vi "ExecuteMenuCommand.vi"(0 "reference":refnum<class "ClassRelationshipEdge.lvclass">, 1 "Command":string, 5 "error in (no error)":errorcluster) -> (14 "reference out":refnum<class "ClassRelationshipEdge.lvclass">, 15 "EditorAction":T1, 19 "error out":errorcluster)   [LabVIEW 2016, in "ClassRelationshipEdge.lvclass"]
uses:
  <resource>/Framework/Providers/Open_GDS/UML/ClassRelationshipEdge_class/ClassRelationshipEdge.lvclass
  <resource>/Framework/Providers/Open_GDS/UML/UMLEditor/UMLEditor EditorActionType.ctl
  <resource>/Framework/Providers/Open_GDS/UML/BentStyle_class/BentStyleType.ctl
  <resource>/Framework/Providers/Open_GDS/UML/BentStyle_class/BentStyle.lvclass
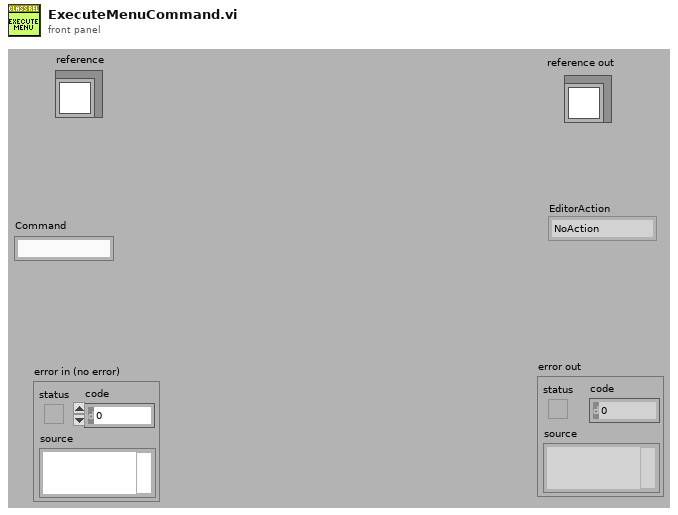
[diagram p1: front panel]
types:
  T1 = typedef "UMLEditor EditorActionType.ctl" = enum16{"NoAction", "Repaint", "ExecuteCommand"}
  T2 = typedef "BentStyle.lvclass/BentStyleType.ctl" = enum16{"STRAIGHT", "HV", "VH", "HVH", "VHV", "ARC"}
  T3 = typedef "ClassRelationshipEdge.lvclass/ObjectAttributes.ctl" = cluster{"bentStyleRef":refnum<class "BentStyle.lvclass">, "startConnectionOffset":cluster{"x":i32, "y":i32}, "endConnectionOffset":cluster{"x":i32, "y":i32}, "MidLineOffset":cluster{"x":i32, "y":i32}, "DepClass":T4}
  T4 = typedef "ReversedEngineering_ViDependencyDetailsType.ctl" = cluster{"ThisVIs/Ctls":path[], "Dependent_VIs/Ctls":path[]}
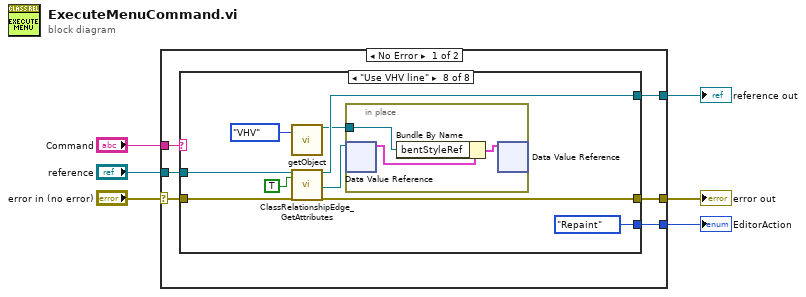
[diagram p0: block diagram]
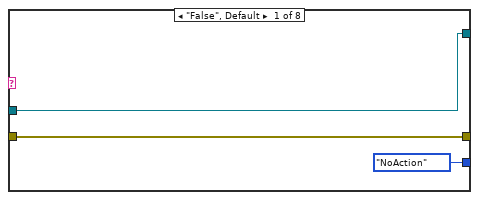
[diagram p2: hidden frame]
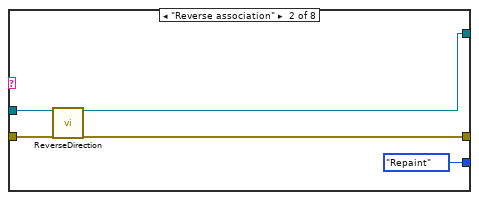
[diagram p3: hidden frame]
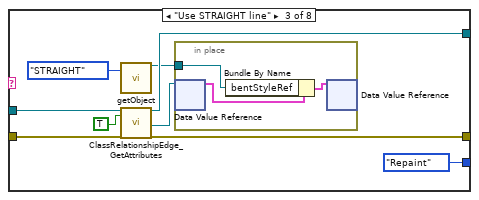
[diagram p4: hidden frame]
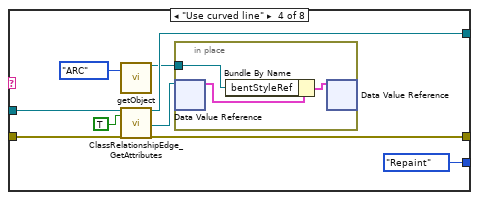
[diagram p5: hidden frame]
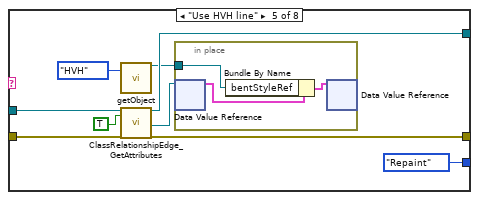
[diagram p6: hidden frame]
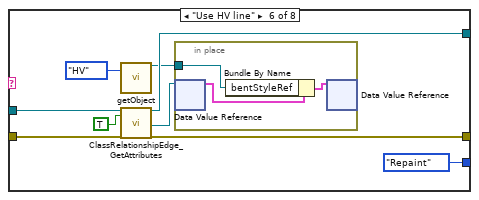
[diagram p7: hidden frame]
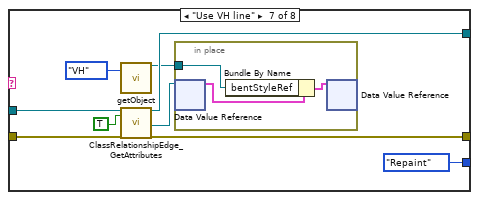
[diagram p8: hidden frame]
diagram:
  n1 = case shown="No Error" "error in (no error)" {
    selector: "error in (no error)" -> [w10 w93]
    tunnel: "reference" -> [w11 w94]
    tunnel: [w9 w93] -> w4
    tunnel: [w7 w94] -> w3
    tunnel: [w8 _] -> w2
    tunnel: "Command" -> [w12 _]
    frame No Error {
      n2 = case shown="\"Use VHV line\"" w12 {
        tunnel: w11 -> [w13 w20 w28 w40 w52 w64 w76 w88]
        tunnel: w10 -> [w14 w19 w27 w39 w51 w63 w75 w87]
        tunnel: [w14 w18 w26 w38 w50 w62 w74 w86] -> w9
        tunnel: [UMLEditor_EditorActionType."NoAction" ("EditorAction") UMLEditor_EditorActionType."Repaint" ("EditorAction") UMLEditor_EditorActionType."Repaint" ("EditorAction") UMLEditor_EditorActionType."Repaint" ("EditorAction") UMLEditor_EditorActionType."Repaint" ("EditorAction") UMLEditor_EditorActionType."Repaint" ("EditorAction") UMLEditor_EditorActionType."Repaint" ("EditorAction") UMLEditor_EditorActionType."Repaint" ("EditorAction")] -> w8
        tunnel: [w13 w16 w25 w37 w49 w61 w73 w85] -> w7
        frame "False", Default {
        }
        frame "Reverse association" {
          n3 = call-dynamic "ReverseDirection.vi"("reference"=w20, "error in (no error)"=w19) -> ("reference out"=w16:refnum<class "ClassRelationshipEdge.lvclass">, "error out"=w18:errorcluster)  [unwired: 16 in]
        }
        frame "Use STRAIGHT line" {
          n4 = call <resource>:"getObject.vi"("bentStyle"=BentStyleType."STRAIGHT") -> ("reference out"=w21:refnum<class "BentStyle.lvclass">)  [unwired: 1 in, 17 out]
          n5 = call <resource>:"ClassRelationshipEdge_GetAttributes.vi"("reference in"=w28, "OnlyGetDvrReference(False)"=TRUE, "error in (no error)"=w27) -> ("reference out"=w25:refnum<class "ClassRelationshipEdge.lvclass">, "DataRef"=w22:refnum<data-value>, "error out"=w26:errorcluster)  [unwired: 13 in, 1 out]
          n6 = in-place {
            in-place-border: w21 -> [w31]
            n7 = in-place-dvr #1(w22) -> (w32:T3)  [unwired: 1 out]
            n8 = Bundle By Name(cluster=w32, "bentStyleRef"=w31) -> (w30:T3)
            n9 = in-place-dvr #1(w30) -> ()  [unwired: 2 out]
          }
        }
        frame "Use curved line" {
          n10 = call <resource>:"getObject.vi"("bentStyle"=BentStyleType."ARC") -> ("reference out"=w33:refnum<class "BentStyle.lvclass">)  [unwired: 1 in, 17 out]
          n11 = call <resource>:"ClassRelationshipEdge_GetAttributes.vi"("reference in"=w40, "OnlyGetDvrReference(False)"=TRUE, "error in (no error)"=w39) -> ("reference out"=w37:refnum<class "ClassRelationshipEdge.lvclass">, "DataRef"=w34:refnum<data-value>, "error out"=w38:errorcluster)  [unwired: 13 in, 1 out]
          n12 = in-place {
            in-place-border: w33 -> [w43]
            n13 = in-place-dvr #2(w34) -> (w44:T3)  [unwired: 1 out]
            n14 = Bundle By Name(cluster=w44, "bentStyleRef"=w43) -> (w42:T3)
            n15 = in-place-dvr #2(w42) -> ()  [unwired: 2 out]
          }
        }
        frame "Use HVH line" {
          n16 = call <resource>:"getObject.vi"("bentStyle"=BentStyleType."HVH") -> ("reference out"=w45:refnum<class "BentStyle.lvclass">)  [unwired: 1 in, 17 out]
          n17 = call <resource>:"ClassRelationshipEdge_GetAttributes.vi"("reference in"=w52, "OnlyGetDvrReference(False)"=TRUE, "error in (no error)"=w51) -> ("reference out"=w49:refnum<class "ClassRelationshipEdge.lvclass">, "DataRef"=w46:refnum<data-value>, "error out"=w50:errorcluster)  [unwired: 13 in, 1 out]
          n18 = in-place {
            in-place-border: w45 -> [w55]
            n19 = in-place-dvr #3(w46) -> (w56:T3)  [unwired: 1 out]
            n20 = Bundle By Name(cluster=w56, "bentStyleRef"=w55) -> (w54:T3)
            n21 = in-place-dvr #3(w54) -> ()  [unwired: 2 out]
          }
        }
        frame "Use HV line" {
          n22 = call <resource>:"getObject.vi"("bentStyle"=BentStyleType."HV") -> ("reference out"=w57:refnum<class "BentStyle.lvclass">)  [unwired: 1 in, 17 out]
          n23 = call <resource>:"ClassRelationshipEdge_GetAttributes.vi"("reference in"=w64, "OnlyGetDvrReference(False)"=TRUE, "error in (no error)"=w63) -> ("reference out"=w61:refnum<class "ClassRelationshipEdge.lvclass">, "DataRef"=w58:refnum<data-value>, "error out"=w62:errorcluster)  [unwired: 13 in, 1 out]
          n24 = in-place {
            in-place-border: w57 -> [w67]
            n25 = in-place-dvr #4(w58) -> (w68:T3)  [unwired: 1 out]
            n26 = Bundle By Name(cluster=w68, "bentStyleRef"=w67) -> (w66:T3)
            n27 = in-place-dvr #4(w66) -> ()  [unwired: 2 out]
          }
        }
        frame "Use VH line" {
          n28 = call <resource>:"getObject.vi"("bentStyle"=BentStyleType."VH") -> ("reference out"=w69:refnum<class "BentStyle.lvclass">)  [unwired: 1 in, 17 out]
          n29 = call <resource>:"ClassRelationshipEdge_GetAttributes.vi"("reference in"=w76, "OnlyGetDvrReference(False)"=TRUE, "error in (no error)"=w75) -> ("reference out"=w73:refnum<class "ClassRelationshipEdge.lvclass">, "DataRef"=w70:refnum<data-value>, "error out"=w74:errorcluster)  [unwired: 13 in, 1 out]
          n30 = in-place {
            in-place-border: w69 -> [w79]
            n31 = in-place-dvr #5(w70) -> (w80:T3)  [unwired: 1 out]
            n32 = Bundle By Name(cluster=w80, "bentStyleRef"=w79) -> (w78:T3)
            n33 = in-place-dvr #5(w78) -> ()  [unwired: 2 out]
          }
        }
        frame "Use VHV line" {
          n34 = call <resource>:"getObject.vi"("bentStyle"=BentStyleType."VHV") -> ("reference out"=w81:refnum<class "BentStyle.lvclass">)  [unwired: 1 in, 17 out]
          n35 = call <resource>:"ClassRelationshipEdge_GetAttributes.vi"("reference in"=w88, "OnlyGetDvrReference(False)"=TRUE, "error in (no error)"=w87) -> ("reference out"=w85:refnum<class "ClassRelationshipEdge.lvclass">, "DataRef"=w82:refnum<data-value>, "error out"=w86:errorcluster)  [unwired: 13 in, 1 out]
          n36 = in-place {
            in-place-border: w81 -> [w91]
            n37 = in-place-dvr #6(w82) -> (w92:T3)  [unwired: 1 out]
            n38 = Bundle By Name(cluster=w92, "bentStyleRef"=w91) -> (w90:T3)
            n39 = in-place-dvr #6(w90) -> ()  [unwired: 2 out]
          }
        }
      }
    }
    frame Error {
    }
  }
  "reference out" <- w3
  "error out" <- w4
  "EditorAction" <- w2
